vi "Set Angle.vi"(6 "Axis":T1, 8 "error in (no error)":errorcluster, 9 "Rate (°/min)":dbl, 10 "Angle (°)":dbl, 11 "Instrument.Cryostat in":refnum<class "Instrument.Cryostat.lvclass">) -> (0 "error out":errorcluster, 3 "Instrument.Cryostat out":refnum<class "Instrument.Cryostat.lvclass">)   [LabVIEW 2019, in "Instrument.Cryostat.lvclass"]
uses:
  Instrument.Cryostat.lvclass
  Typedefs/Rotator Axis--Enum.ctl
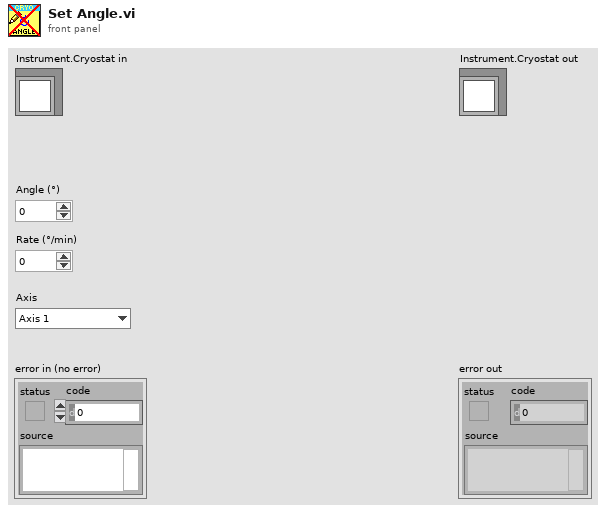
[diagram p1: front panel]
types:
  T1 = typedef "Instrument.Cryostat.lvclass/Rotator Axis--Enum.ctl" = enum16{"Axis 1", "Axis 2"}
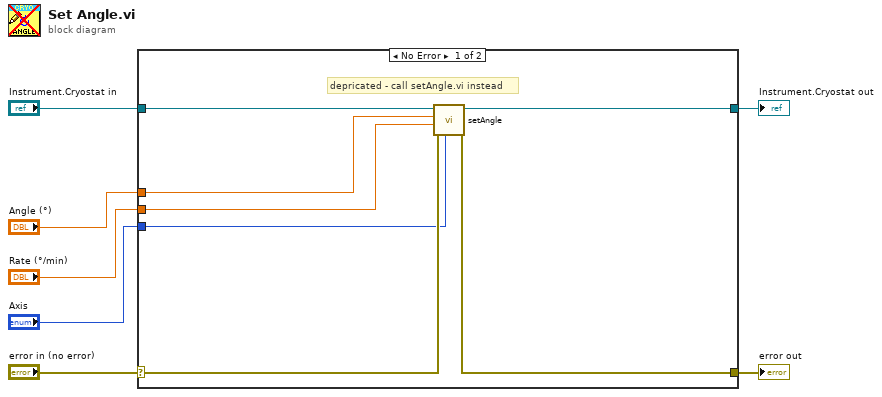
[diagram p0: block diagram]
diagram:
  n1 = case shown="No Error" "error in (no error)" {
    selector: "error in (no error)" -> [w12 w16]
    tunnel: [w11 w16] -> w6
    tunnel: [w14 w15] -> w4
    tunnel: "Instrument.Cryostat in" -> [w13 w15]
    tunnel: "Angle (°)" -> [w8 _]
    tunnel: "Rate (°/min)" -> [w9 _]
    tunnel: "Axis" -> [w10 _]
    frame No Error {
      # "depricated - call setAngle.vi instead"
      n2 = call-dynamic "setAngle.vi"("Channel"=w10, "error in (no error)"=w12, "Rate (°/min)"=w9, "Angle (°)"=w8, "Instrument.Cryostat in"=w13) -> ("error out"=w11:errorcluster, "Instrument.Cryostat out"=w14:refnum<class "Instrument.Cryostat.lvclass">)  [unwired: 5 in]
    }
    frame Error {
    }
  }
  "error out" <- w6
  "Instrument.Cryostat out" <- w4
